vi "Contour Integral.vi"(6 "Reverse direction?":bool, 7 "Method":enum16{"Trapezium Rule", "Simpson's Rule"}(ring), 10 "Y":dbl[](array[numeric]), 11 "X":dbl[](array[numeric])) -> (3 "Integral of Y":dbl)   [LabVIEW 2022 SP3]
panel:
  out "XY Graph":cluster{"X":dbl[], "Y":dbl[]}(graph)
  out "Array":dbl[](array[numeric])
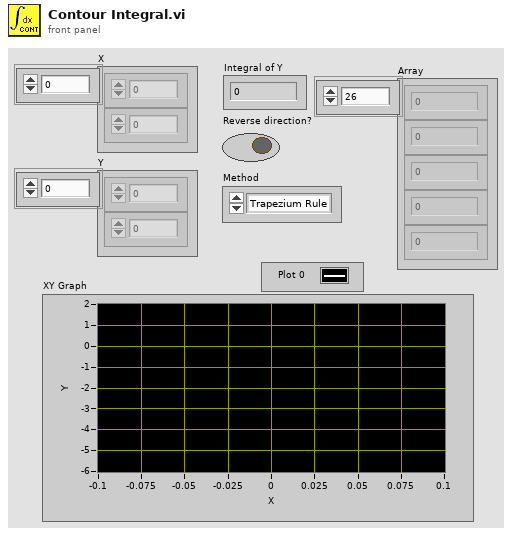
[diagram p1: front panel]
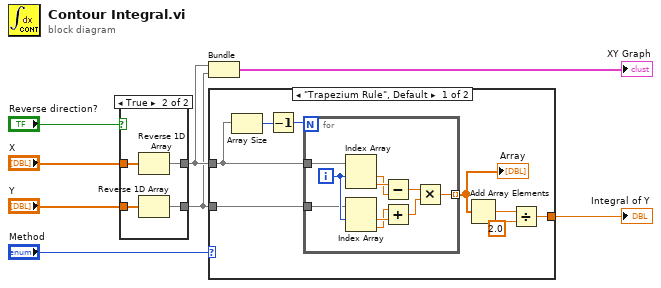
[diagram p0: block diagram]
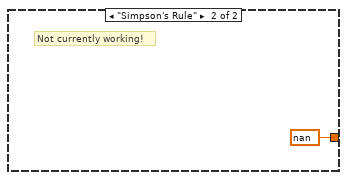
[diagram p3: hidden frame]
diagram:
  n1 = case shown="True" "Reverse direction?" {
    tunnel: [w10 w12] -> w3
    tunnel: "X" -> [w10 w14]
    tunnel: [w9 w11] -> w2
    tunnel: "Y" -> [w9 w13]
    frame False {
    }
    frame True {
      n2 = Reverse 1D Array(array=w14) -> (reversed array=w12:dbl[])
      n3 = Reverse 1D Array(array=w13) -> (reversed array=w11:dbl[])
    }
  }
  n4 = Bundle("X"=w3, "Y"=w2) -> (→"XY Graph":cluster{"X":dbl[], "Y":dbl[]})  [unwired: 1 in]
  n5 = case shown="\"Trapezium Rule\", Default" "Method" {
    tunnel: w2 -> [w22 _]
    tunnel: w3 -> [w17 _]
    tunnel: [w18 nan] -> w8
    frame "Trapezium Rule", Default {
      n6 = Array Size(array=w17) -> (size(s)=w15:i32)
      n7 = Decrement(x=w15) -> (x-1=w16:i32)
      n8 = for {
        N: w16 -> [_]
        tunnel: w17 -> [w24]
        tunnel: w22 -> [w23]
        tunnel: [w28] -> w19 mode=indexing
        i -> [w32]
        n9 = Index Array(array=w24, index #1=w32) -> (element #1=w30:dbl, element #2=w31:dbl)  [unwired: 1 in]
        n10 = Index Array(array=w23, index #1=w32) -> (element #1=w26:dbl, element #2=w25:dbl)  [unwired: 1 in]
        n11 = Subtract(x=w31, y=w30) -> (x-y=w29:dbl)
        n12 = Add(x=w25, y=w26) -> (x+y=w27:dbl)
        n13 = Multiply(x=w29, y=w27) -> (x*y=w28:dbl)
      }
      "Array" <- w19
      n14 = Add Array Elements(numeric array=w19) -> (sum=w21:dbl)
      n15 = Divide(x=w21, y=2.0) -> (x/y=w18:dbl)
    }
    frame "Simpson's Rule" {
      # "Not currently working!"
    }
  }
  "Integral of Y" <- w8
